vi "Test REP Socket.vi"(8 "error in (no error)":errorcluster, 11 "RemoteControl.ZMQ in":refnum<class "RemoteControl.ZMQ.lvclass">) -> (0 "error out":errorcluster, 3 "RemoteControl.ZMQ out":refnum<class "RemoteControl.ZMQ.lvclass">)   [LabVIEW 2019, in "RemoteControl.ZMQ.lvlib" / "RemoteControl.ZMQ.lvclass"]
uses:
  RemoteControl.ZMQ.lvclass
  <vilib>/addons/zeromq/zmq_context.lvclass
  <vilib>/addons/_JKI Toolkits/Caraya/classes/Assert/Assert.lvclass
  <vilib>/addons/_JKI Toolkits/Caraya/classes/Assert/Assert Not Error.vi
  <vilib>/addons/zeromq/socket_type.ctl
  <vilib>/addons/zeromq/zeromq.lvlib
  <vilib>/addons/zeromq/zmq_socket.lvclass
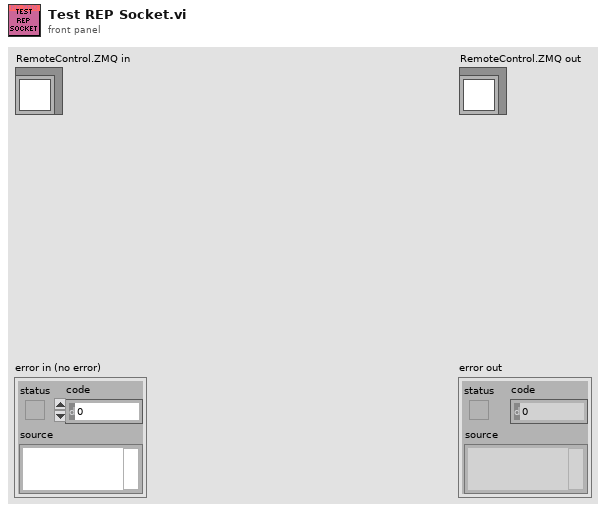
[diagram p1: front panel]
types:
  T1 = typedef "zeromq.lvlib/socket_type.ctl" = enum8{"ZMQ_PAIR", "ZMQ_PUB", "ZMQ_SUB", "ZMQ_REQ", "ZMQ_REP", "ZMQ_DEALER", "ZMQ_ROUTER", "ZMQ_PULL", "ZMQ_PUSH", "ZMQ_XPUB", "ZMQ_XSUB", "ZMQ_STREAM", "ZMQ_SERVER", "ZMQ_CLIENT", "ZMQ_RADIO", "ZMQ_DISH", "ZMQ_GATHER", "ZMQ_SCATTER", "ZMQ_DGRAM"}
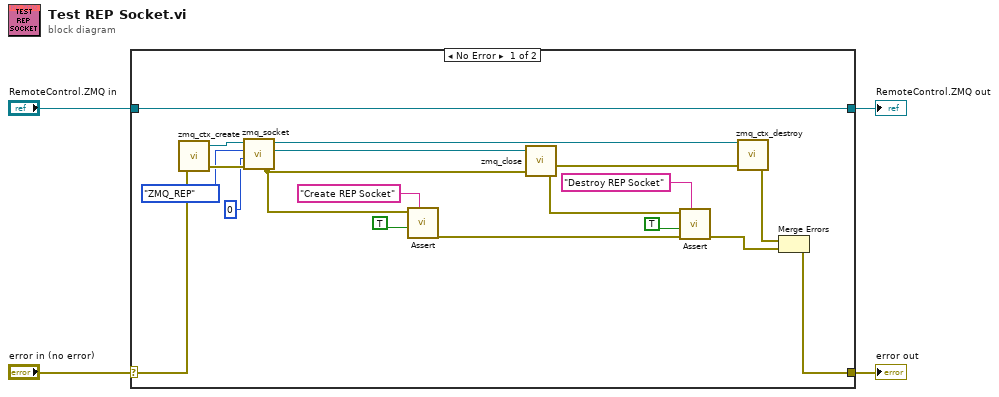
[diagram p0: block diagram]
diagram:
  n1 = case shown="No Error" "error in (no error)" {
    selector: "error in (no error)" -> [w21 w24]
    tunnel: [w5 w24] -> w3
    tunnel: [w14 w23] -> w1
    tunnel: "RemoteControl.ZMQ in" -> [w14 w23]
    frame No Error {
      n2 = call <vilib>:"zmq_ctx_create.vi"("error in"=w21) -> ("error out"=w18:errorcluster, "context out"=w19:refnum<class "zmq_context.lvclass">)  [unwired: 3 in]
      n3 = call <vilib>:"zmq_socket.vi"("error in"=w18, "linger (ms)"=0, "socket type"=socket_type."ZMQ_REP", "context in"=w19) -> ("error out"=w9:errorcluster, "socket out"=w15:refnum<class "zmq_socket.lvclass">, "context out"=w13:refnum<class "zmq_context.lvclass">)  [unwired: 1 in]
      n4 = call-poly <vilib>:"Assert.vi"("Label"="Create REP Socket", "Register with caller test (F)"=TRUE, "Not Error?"=w9) -> ("error out"=w10:errorcluster)  [unwired: 7 in, 1 out]
      n5 = call <vilib>:"zmq_close.vi"("error in"=w9, "socket"=w15) -> ("error out"=w8:errorcluster)  [unwired: 3 in]
      n6 = call-poly <vilib>:"Assert.vi"("Label"="Destroy REP Socket", "error in (no error)"=w10, "Register with caller test (F)"=TRUE, "Not Error?"=w8) -> ("error out"=w6:errorcluster)  [unwired: 6 in, 1 out]
      n7 = call <vilib>:"zmq_ctx_destroy.vi"("error in"=w8, "context in"=w13) -> ("error out"=w7:errorcluster)  [unwired: 3 in]
      n8 = Merge Errors(w7, w6) -> (w5:errorcluster)
    }
    frame Error {
    }
  }
  "error out" <- w3
  "RemoteControl.ZMQ out" <- w1
